vi "Add.vi"(9 "B":dbl, 10 "A":dbl) -> (2 "A + B":dbl)   [LabVIEW 2012]
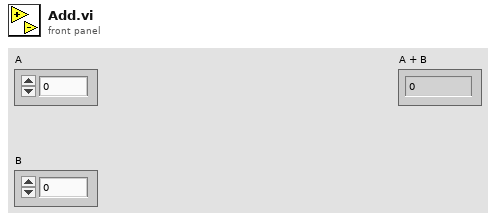
[diagram p1: front panel]
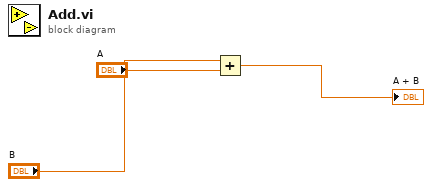
[diagram p0: block diagram]
diagram:
  n1 = Add(x="B", y="A") -> (x+y=→"A + B":dbl)
